vi "PCA9535 - 0x25.vi"(8 "error in (no error)":errorcluster, 11 "handle":u64 format="%x") -> (0 "error out":errorcluster, 2 "0X25 Pass or Fail":bool, 3 "handle 2":u64)   [LabVIEW 2024]
panel:
  out "sizeTransferred (Output) 3":u32
  out "sizeTransferred (Output) 2":u32
  out "sizeTransferred (Output)":u32
  out "p/f1":bool
  out "p/f2":bool
  out "p/f3":bool
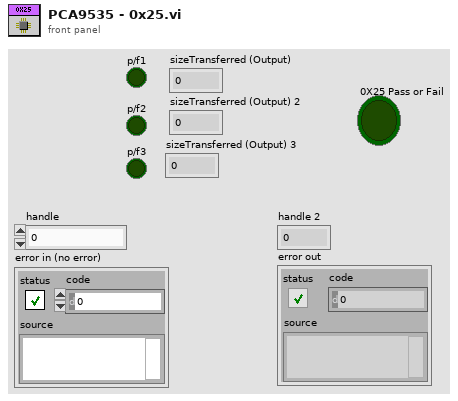
[diagram p1: front panel]
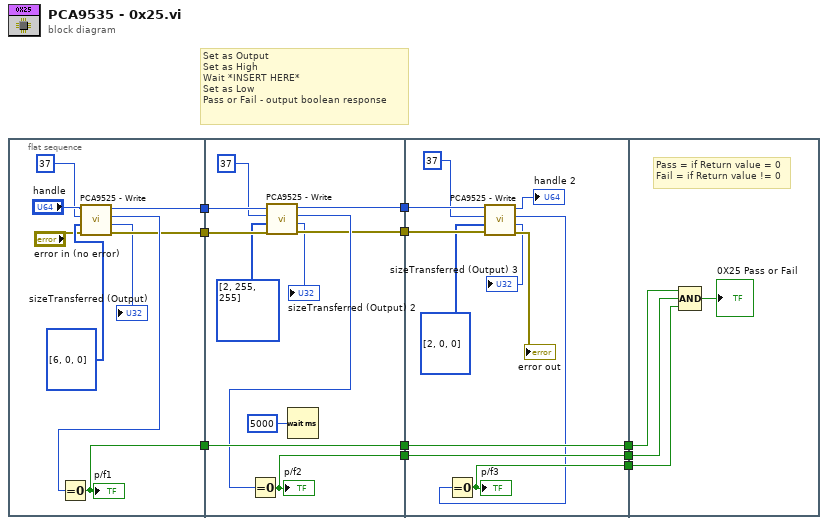
[diagram p0: block diagram]
diagram:
  # "Set as Output \nSet as High\nWait *INSERT HERE*\nSet as Low\nPass or Fail - output boolean response"
  n1 = flat-sequence {
    tunnel: [w19] -> w7
    tunnel: [w17] -> w4
    tunnel: [w15] -> w2
    tunnel: [w29] -> w9
    tunnel: w7 -> [w28]
    tunnel: [w28] -> w6
    tunnel: w4 -> [w26]
    tunnel: [w25] -> w3
    tunnel: w2 -> [w24]
    tunnel: [w23] -> w1
    tunnel: [w41] -> w10
    tunnel: w9 -> [w40]
    tunnel: [w40] -> w8
    tunnel: w6 -> [w39]
    tunnel: [w39] -> w5
    tunnel: w3 -> [w38]
    tunnel: w1 -> [w34]
    tunnel: w10 -> [w45]
    tunnel: w8 -> [w44]
    tunnel: w5 -> [w43]
    frame #0 {
      n2 = call "PCA9525 - Write.vi"("error in (no error)"="error in (no error)", "buffer"=u8[] [6, 0, 0], "deviceAddress"=u8 37, "handle"="handle") -> ("error out"=w15:errorcluster, "sizeTransferred (Output)"=→"sizeTransferred (Output)":u32, "return (Output)"=w18:u64, "handle 2"=w17:u64)  [unwired: 4 in]
      n3 = Equal To 0?(x=w18) -> (x = 0?=w19:bool)
      "p/f1" <- w19
    }
    frame #1 {
      n4 = call "PCA9525 - Write.vi"("error in (no error)"=w24, "buffer"=u8[] [2, 255, 255], "deviceAddress"=u8 37, "handle"=w26) -> ("error out"=w23:errorcluster, "sizeTransferred (Output)"=→"sizeTransferred (Output) 2":u32, "return (Output)"=w27:u64, "handle 2"=w25:u64)  [unwired: 4 in]
      n5 = Equal To 0?(x=w27) -> (x = 0?=w29:bool)
      "p/f2" <- w29
      n6 = Wait (ms)(milliseconds to wait=u32 5000) -> ()  [unwired: 1 out]
    }
    frame #2 {
      n7 = call "PCA9525 - Write.vi"("error in (no error)"=w34, "buffer"=u8[] [2, 0, 0], "deviceAddress"=u8 37, "handle"=w38) -> ("error out"=→"error out":errorcluster, "sizeTransferred (Output)"=→"sizeTransferred (Output) 3":u32, "return (Output)"=w35:u64, "handle 2"=→"handle 2":u64)  [unwired: 4 in]
      n8 = Equal To 0?(x=w35) -> (x = 0?=w41:bool)
      "p/f3" <- w41
    }
    frame #3 {
      # "Pass = if Return value = 0\nFail = if Return value != 0"
      n9 = Compound Arithmetic op=AND(w43, w44, w45) -> (→"0X25 Pass or Fail":bool)
    }
  }
